vi "channeldata_2ch_interleaved.vi"() -> ()   [LabVIEW 2019]
panel:
  out "Error Out":errorcluster
  in  "TDMS File":path=path "C:/Python/projects/nitdms/tests/tdms_files/channeldata_2ch_interleaved.tdms"
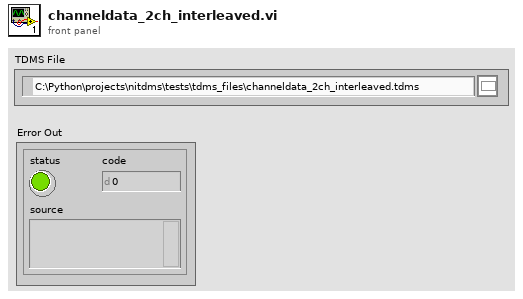
[diagram p1: front panel]
types:
  T1 = enum16{"open", "open or create", "create or replace", "create", "open (read-only)"}
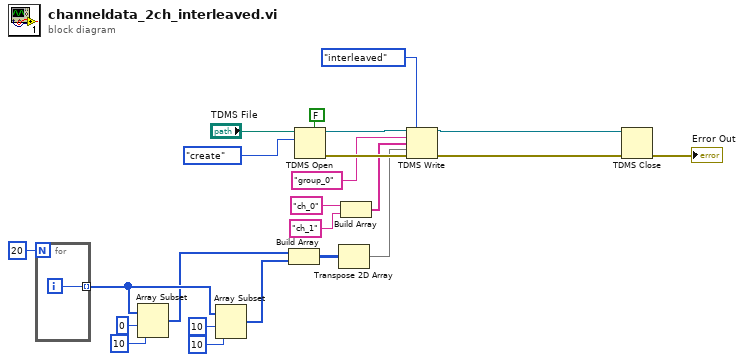
[diagram p0: block diagram]
diagram:
  n1 = for {
    N: 20 -> [_]
    tunnel: [w24] -> w11 mode=indexing
    i -> [w24]
  }
  n2 = Array Subset(array=w11, index=0, length=10) -> (w10:i32[])
  n3 = Array Subset(array=w11, index=10, length=10) -> (w9:i32[])
  n4 = Build Array(w10, w9) -> (w2:i32[][])
  n5 = TDMS Open(5:FALSE ("create index file? (T)"), 10:T1."create" ("operation (0:open)"), 11:"TDMS File") -> (0:w19:errorcluster, 3:w18:refnum<k34>)  [unwired: 4 in]
  n6 = Transpose 2D Array(2D array=w2) -> (transposed array=w1:i32[][])
  n7 = Build Array("ch_0", "ch_1") -> (w6:string[])
  n8 = TDMS Write(0:w18, 1:enum16{"decimated", "interleaved"}."interleaved" ("data layout (0:decimated)"), 5:"group_0", 7:w6, 9:w1, 11:w19) -> (4:w4:refnum<k34>, 15:w5:errorcluster)  [unwired: 2 out]
  n9 = TDMS Close(8:w5, 11:w4) -> (0:→"Error Out":errorcluster)  [unwired: 1 out]
